vi "kD2A Encode.vi"(10 "Position":u8, 11 "Value":i16) -> (3 "Coded Output":u16)   [LabVIEW 2010, in "kevLib2011.lvlib"]
uses:
  kevLib2011.lvlib
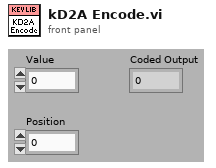
[diagram p1: front panel]
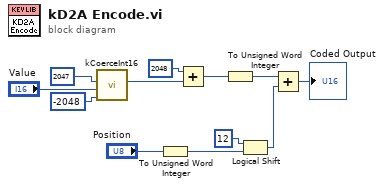
[diagram p0: block diagram]
diagram:
  n1 = call "kCoerceInt16.vi"("lower"=i16 -2048 ("upper"), "input"="Value", "upper"=i16 2047) -> ("output"=w8:i16)  [unwired: 7 in, 1 out]
  n2 = To Unsigned Word Integer(number="Position") -> (unsigned 16bit integer=w2:u16)
  n3 = Add(x=i16 2048, y=w8) -> (x+y=w9:i16)
  n4 = To Unsigned Word Integer(number=w9) -> (unsigned 16bit integer=w10:u16)
  n5 = Logical Shift(y=i8 12, x=w2) -> (x << y=w11:u16)
  n6 = Add(x=w10, y=w11) -> (x+y=→"Coded Output":u16)
